vi "MPU_Stick_Plotter_Core.vi"(0 "Value (original)":dbl, 1 "Time (ms)":dbl, 2 "Offset & Multiplier":T2, 3 "Maximum":dbl, 4 "Minimum":dbl, 5 "error in (no error)":errorcluster, 6 "Channel Name":string, 7 "Plot update interval (ms)":u32=100, 8 "Number of vertical divisions":u16, 9 "Number of horizontal divisions":u16, 10 "Plot reference":refnum<vi>, 11 "Command":T3, 13 "Time axis length (ms)":u32=10000) -> (15 "Sample value":dbl, 16 "Plot Data":T1, 17 "Sample time (ms)":dbl, 19 "error out":errorcluster)   [LabVIEW 2017]
uses:
  Controls/MPU_Stick_Plotter_Core_Commands.ctl
  <vilib>/Utility/miscctls.llb/LVOffsetAndMultiplierTypeDef.ctl
  Controls/MPU_Stick_Plotter_Core_Channel_Data.ctl
  <vilib>/Utility/miscctls.llb/LVPointDoubleTypeDef.ctl
panel:
  in  "Use Internal timer ?":bool
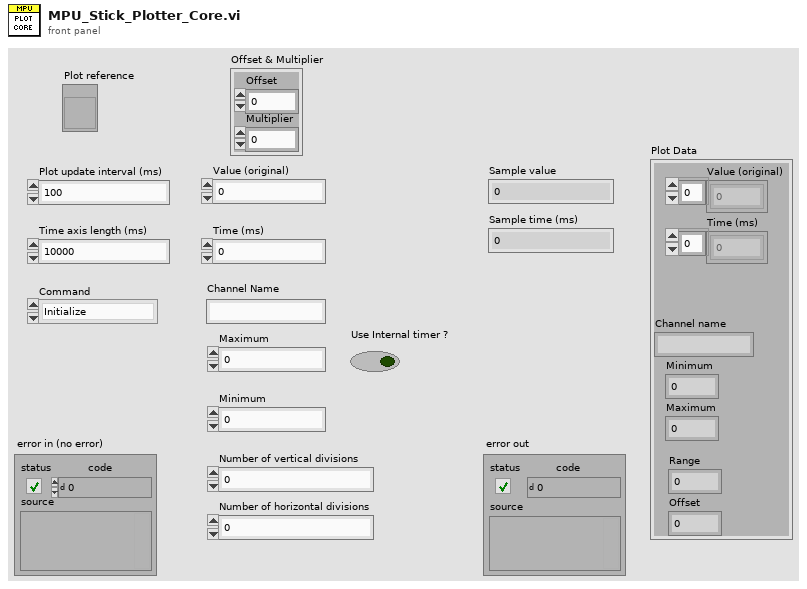
[diagram p1: front panel]
types:
  T1 = typedef "MPU_Stick_Plotter_Core_Channel_Data.ctl" = cluster{"Value (original)":dbl[], "Time (ms)":dbl[], "Channel name":string, "Minimum":dbl, "Maximum":dbl, "Offset":dbl, "Range":dbl}
  T2 = typedef "LVOffsetAndMultiplierTypeDef.ctl" = cluster{"Offset":dbl, "Multiplier":dbl}
  T3 = typedef "MPU_Stick_Plotter_Core_Commands.ctl" = enum16{"Initialize", "Add Channel", "Remove Channel", "Set Channel Minimum Value", "Set Channel Maximum Value", "Set Offset & Multiplier", "Get Offset & Multiplier", "Update Channel", "Get Cursor Data", "Clear", "Reset"}
  T4 = typedef "LVPointDoubleTypeDef.ctl" = cluster{"X":dbl, "Y":dbl}
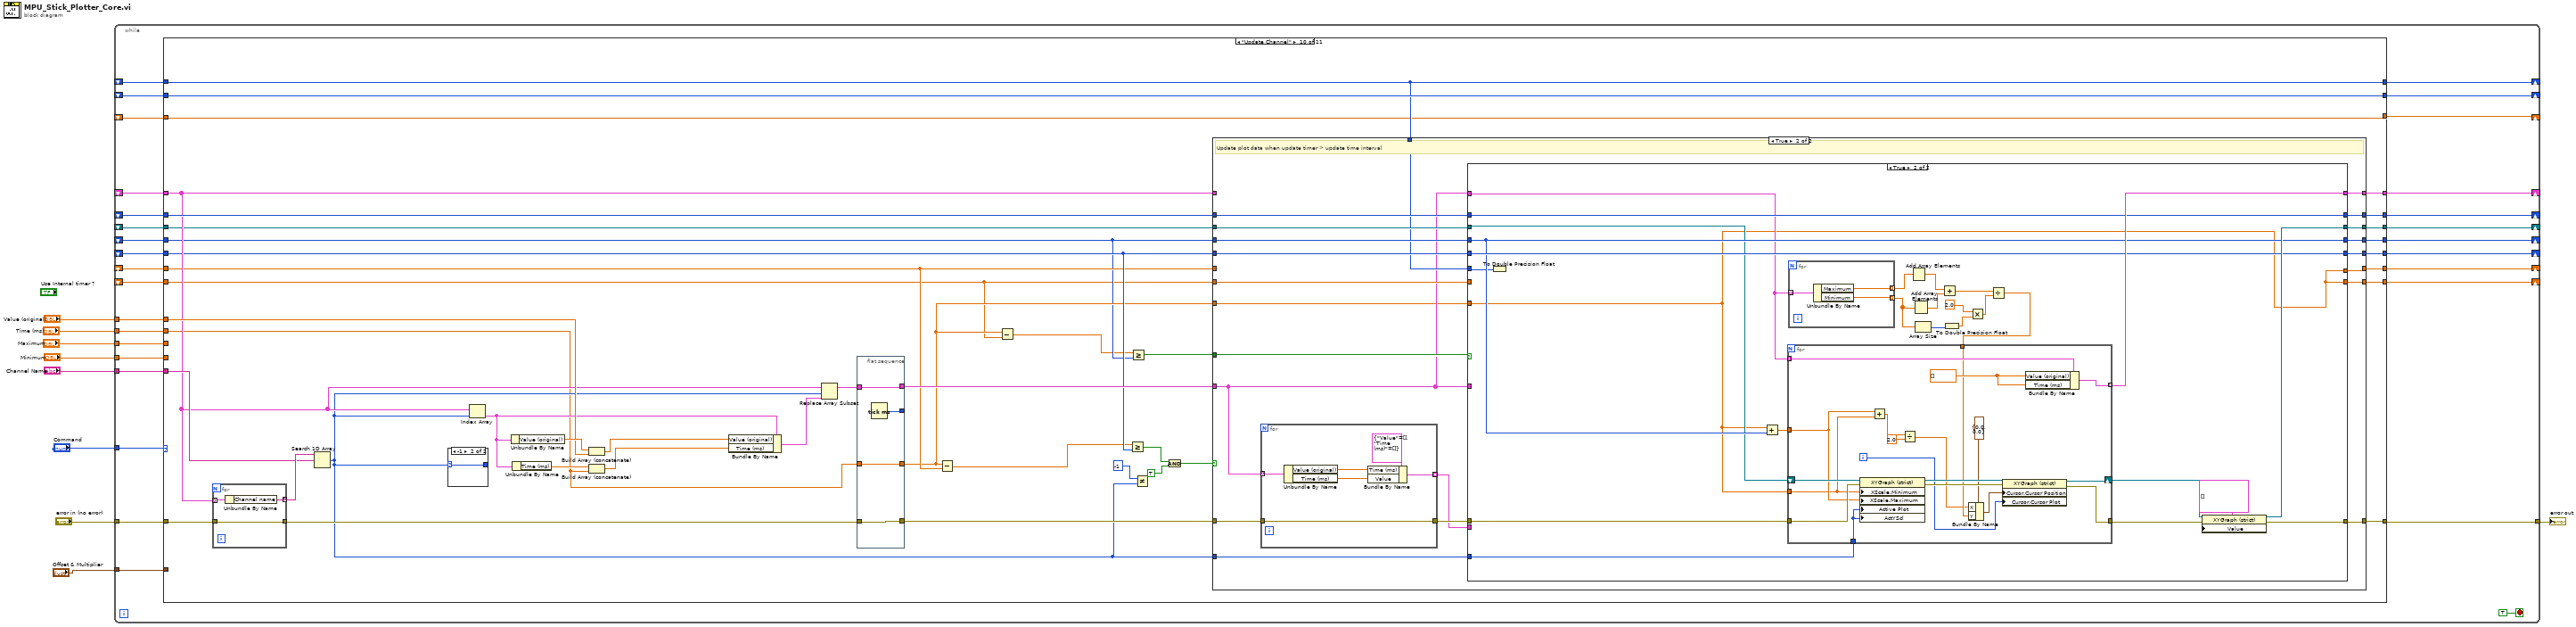
[diagram p0: block diagram]
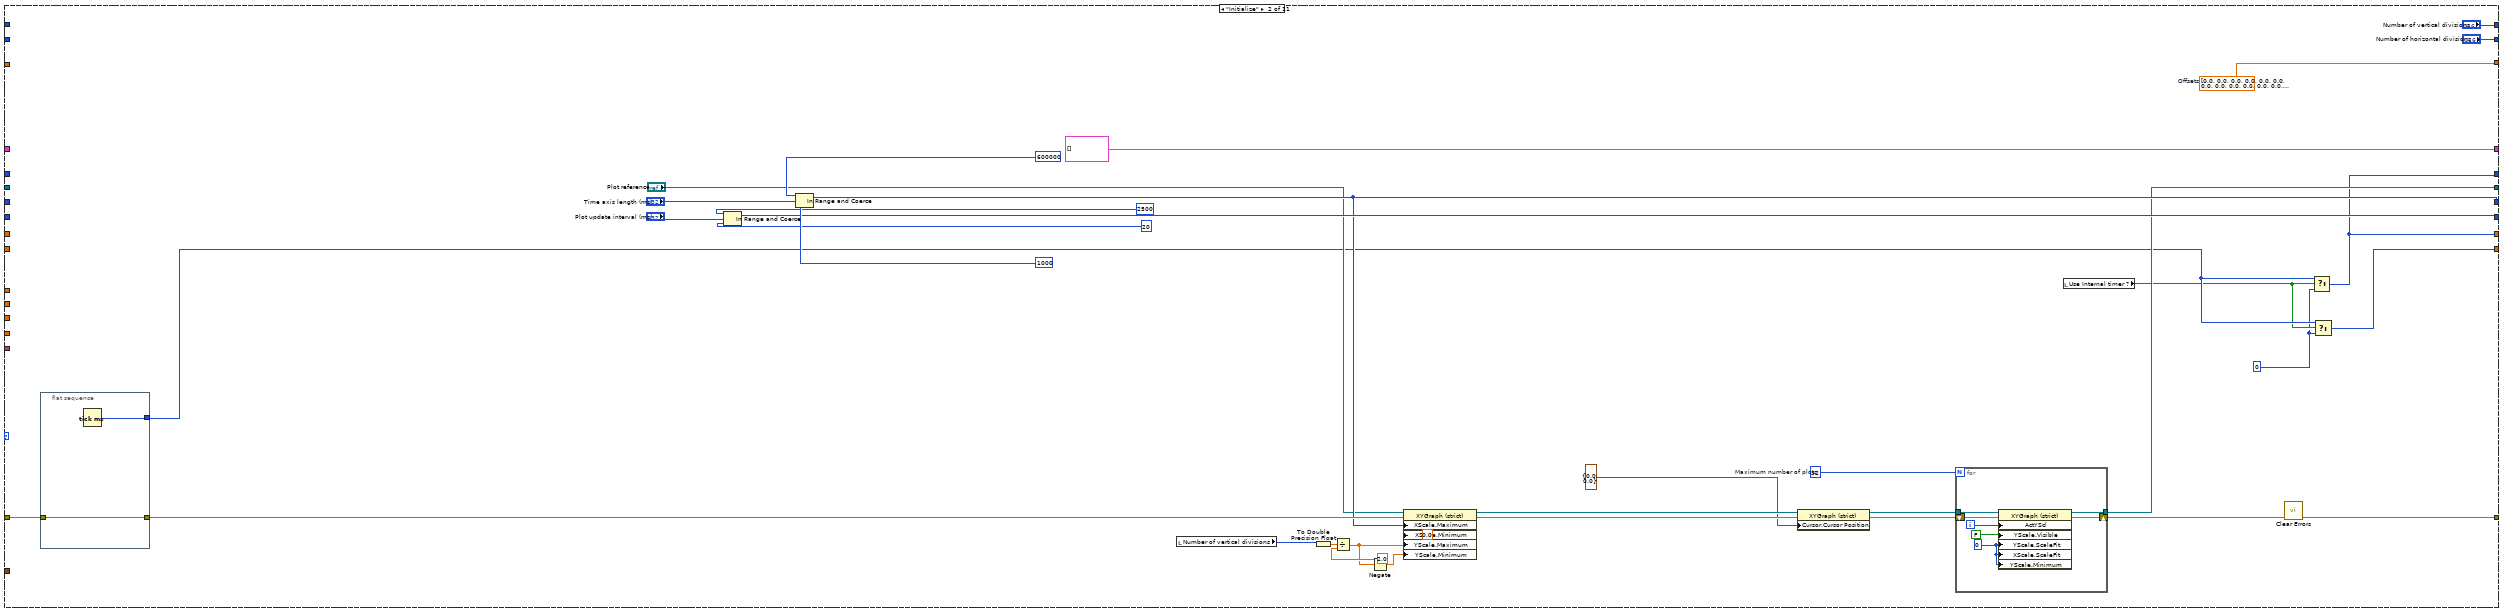
[diagram p3: hidden frame]
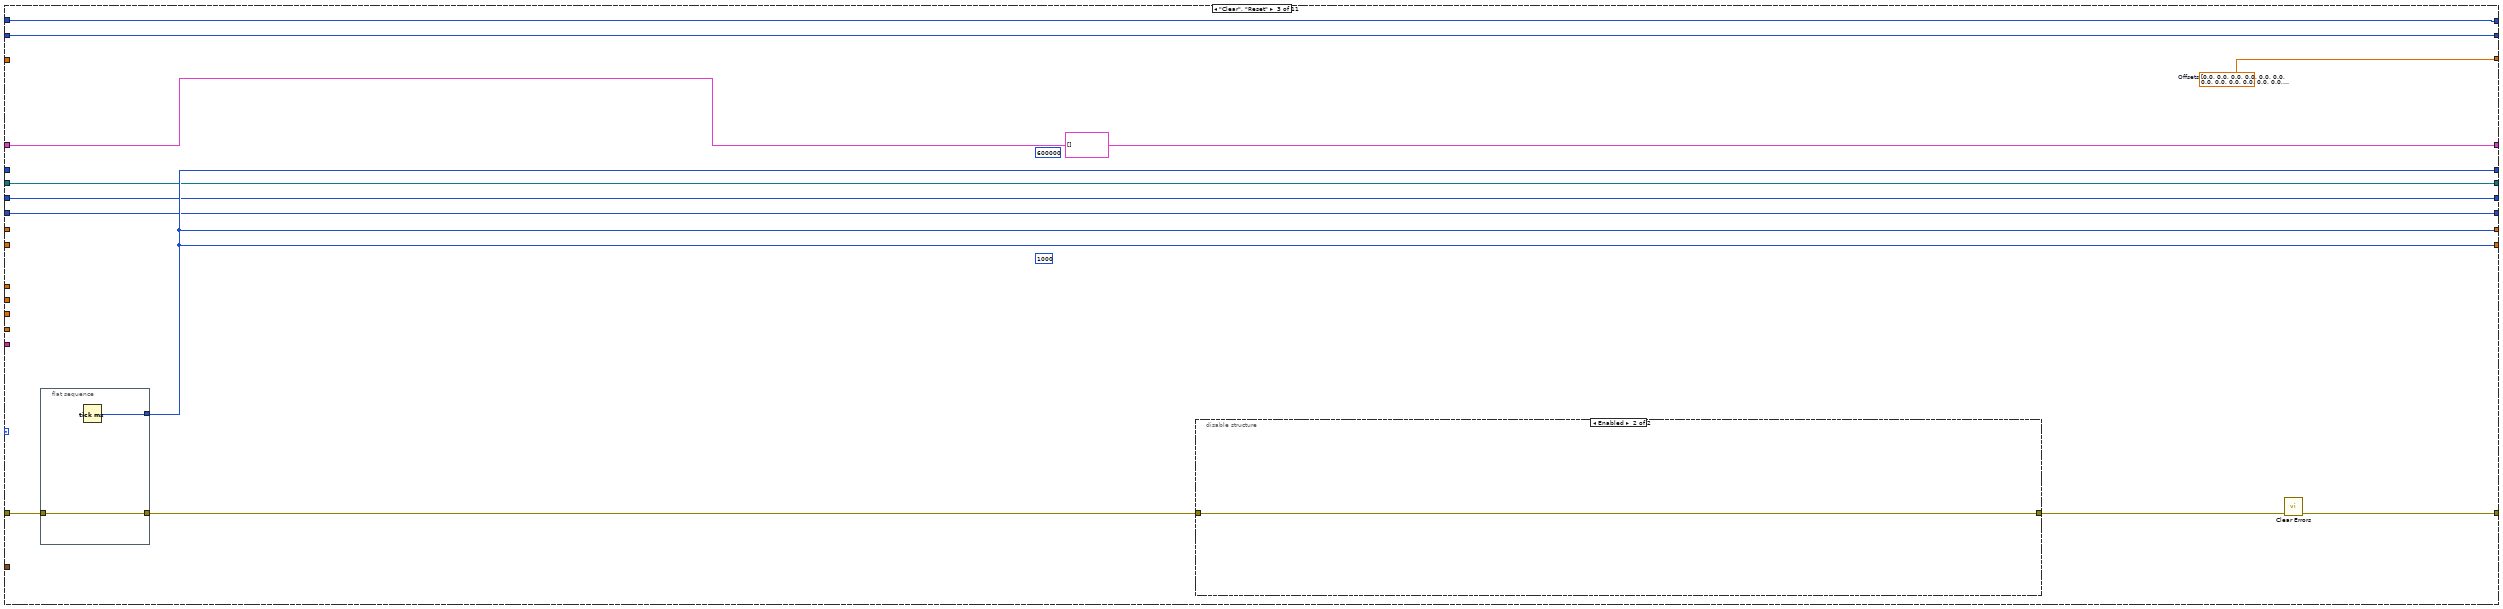
[diagram p4: hidden frame]
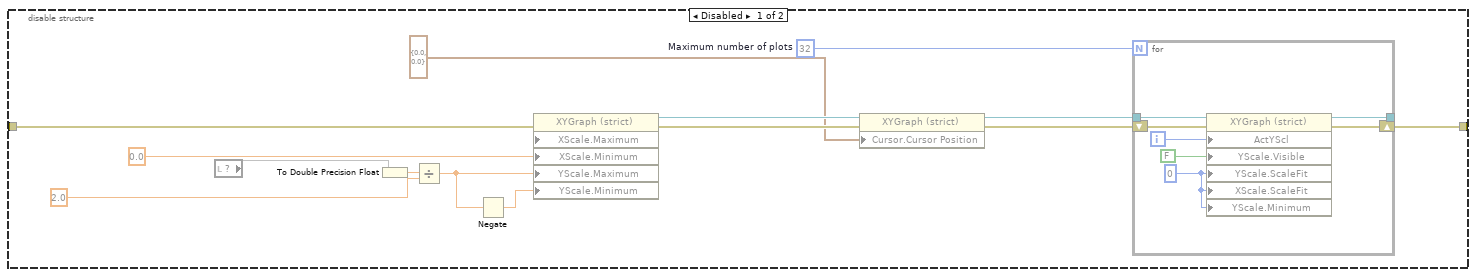
[diagram p5: hidden frame]
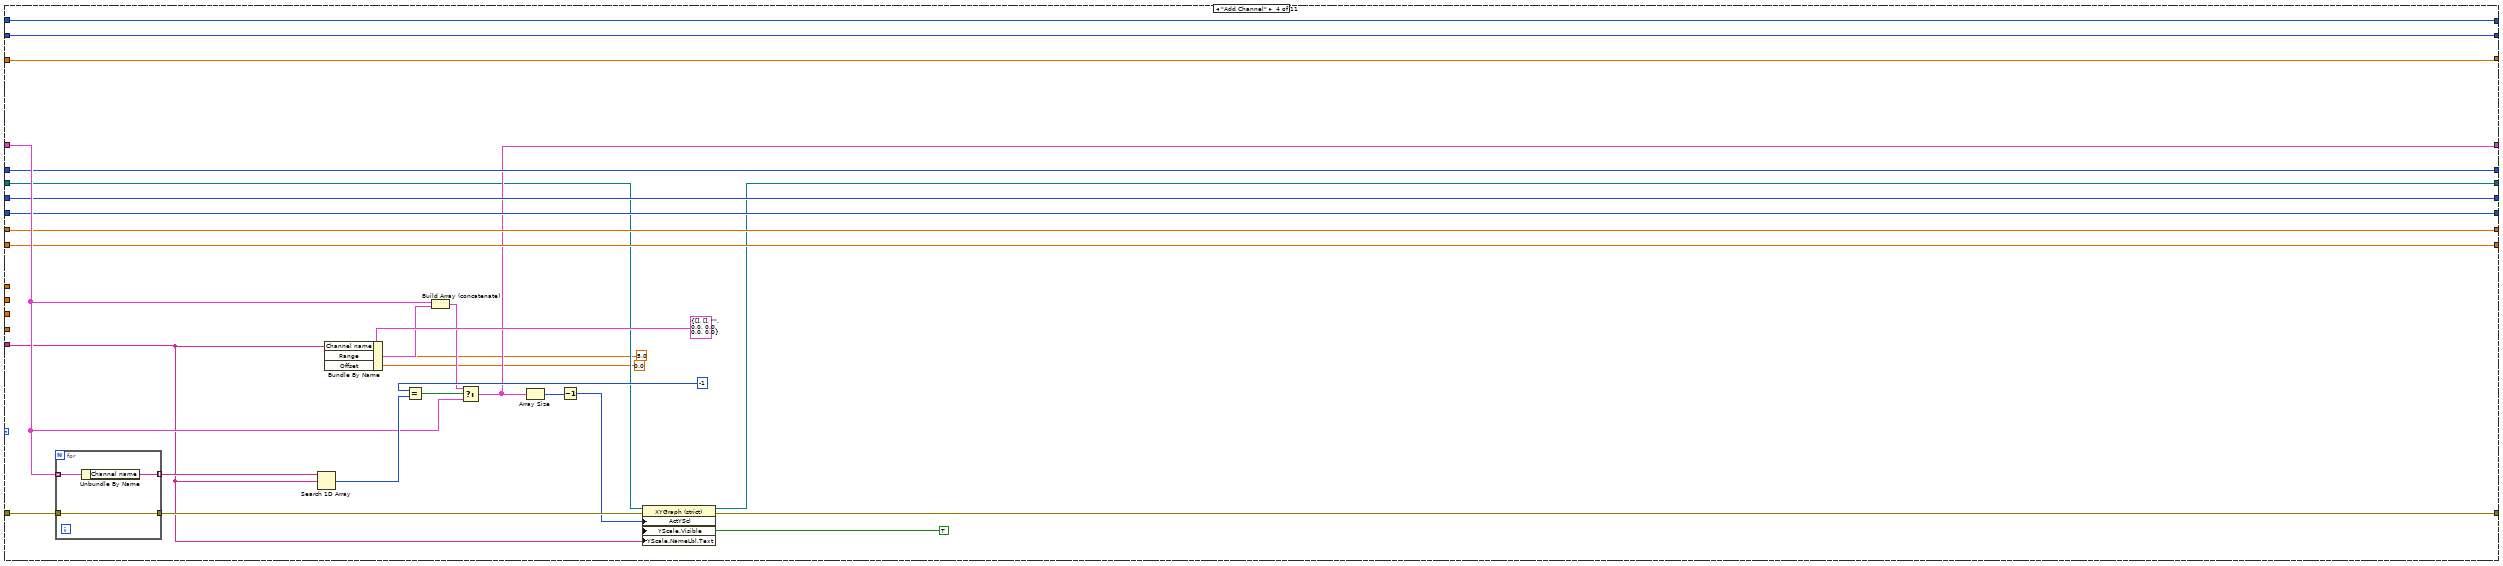
[diagram p6: hidden frame]
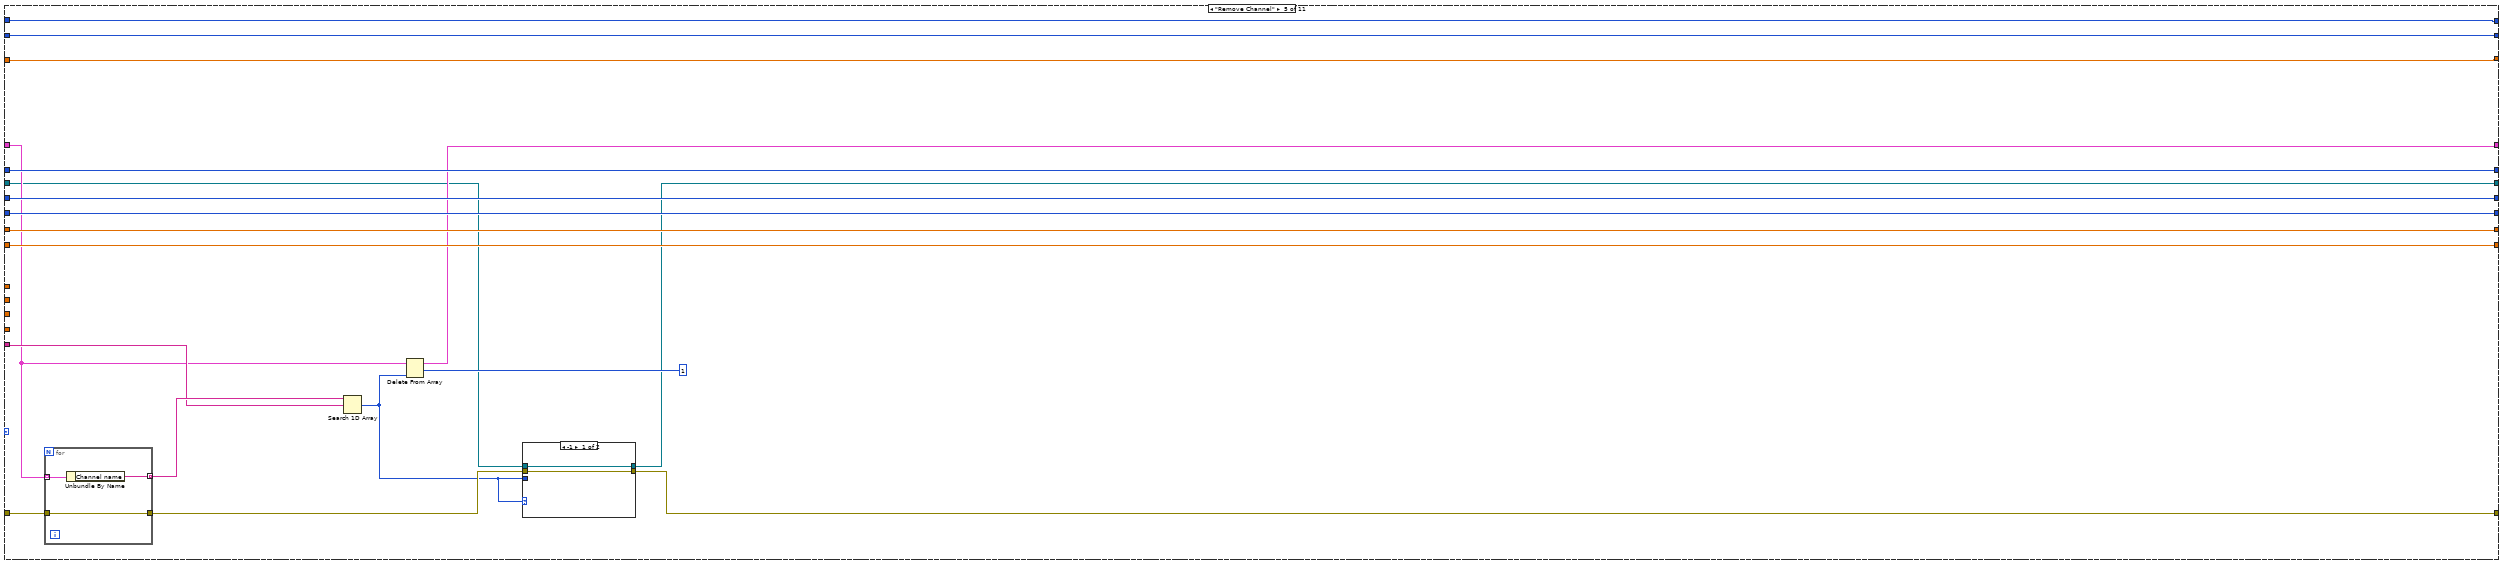
[diagram p7: hidden frame]
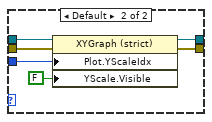
[diagram p8: hidden frame]
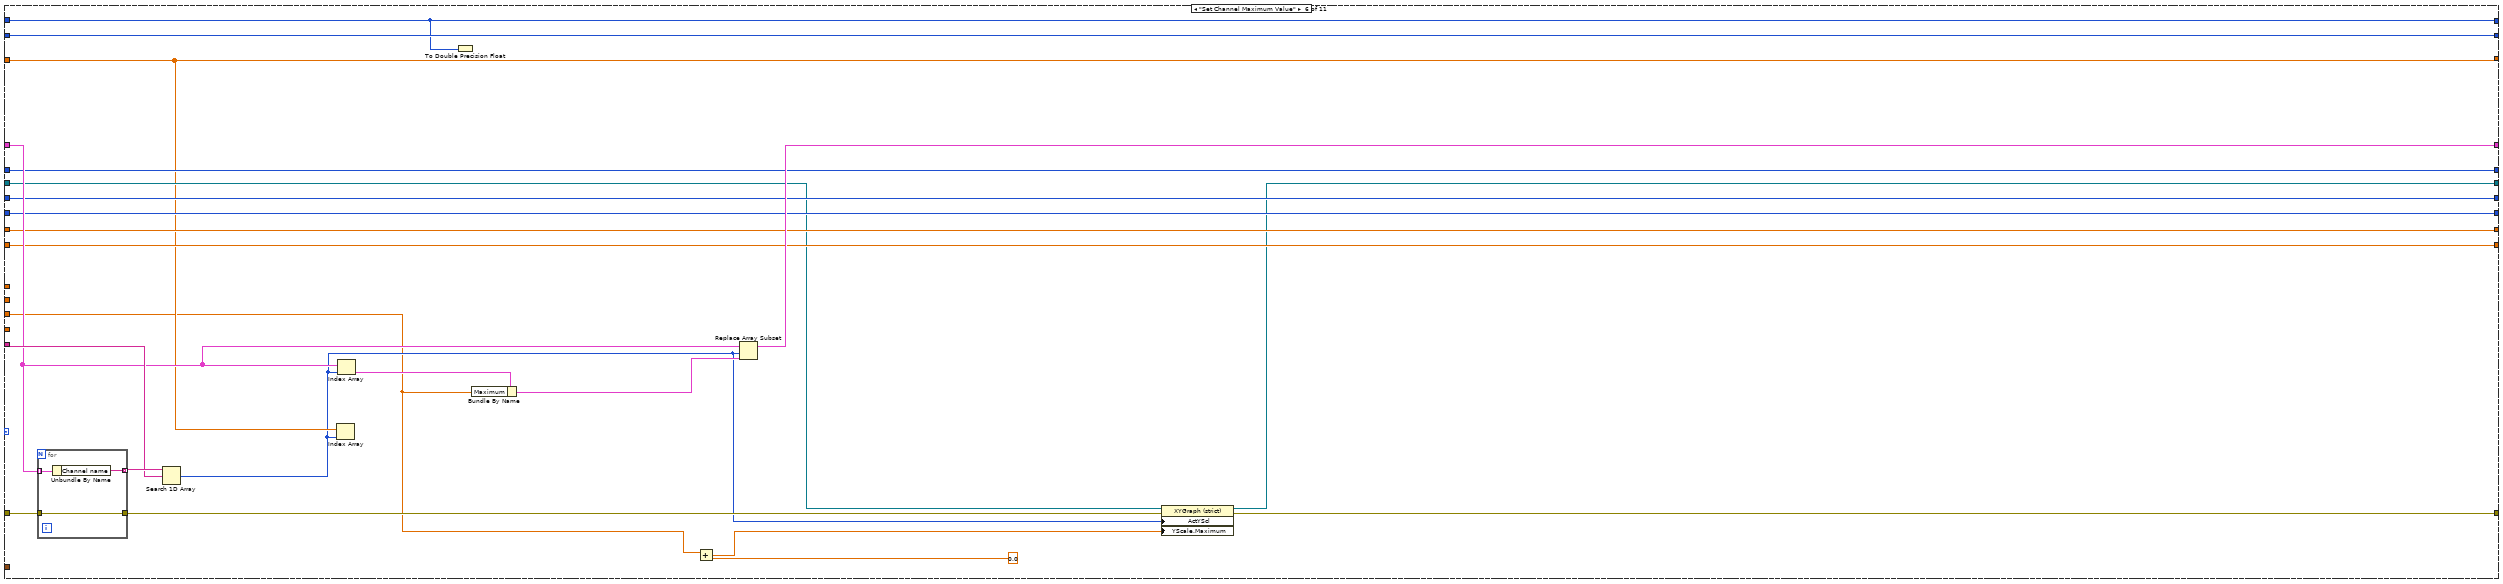
[diagram p9: hidden frame]
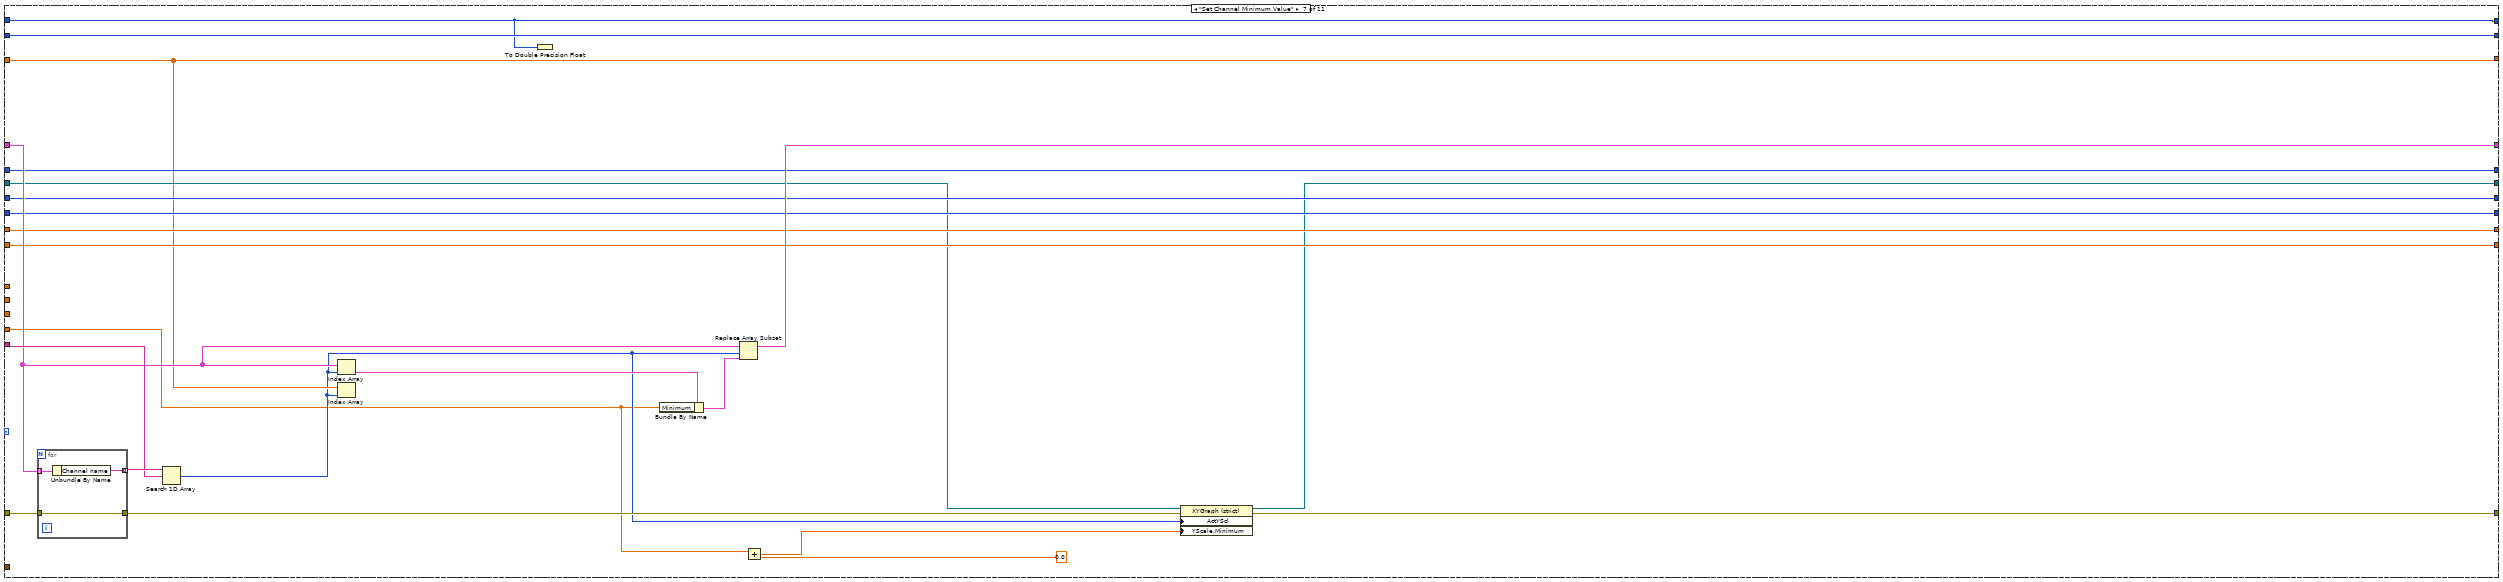
[diagram p10: hidden frame]
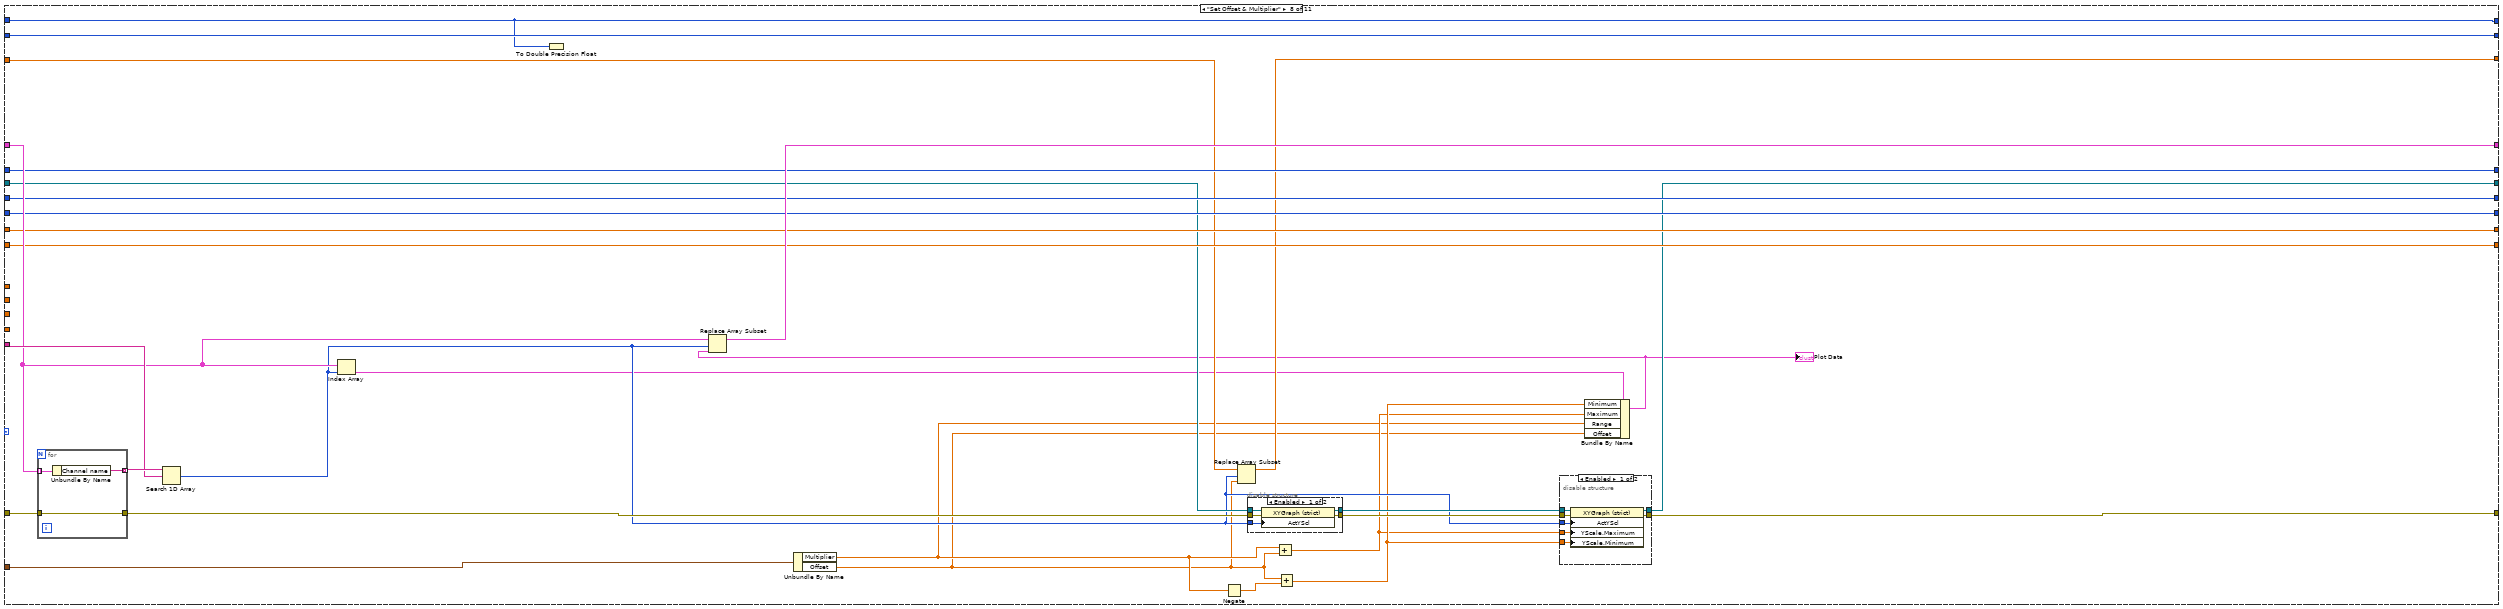
[diagram p11: hidden frame]
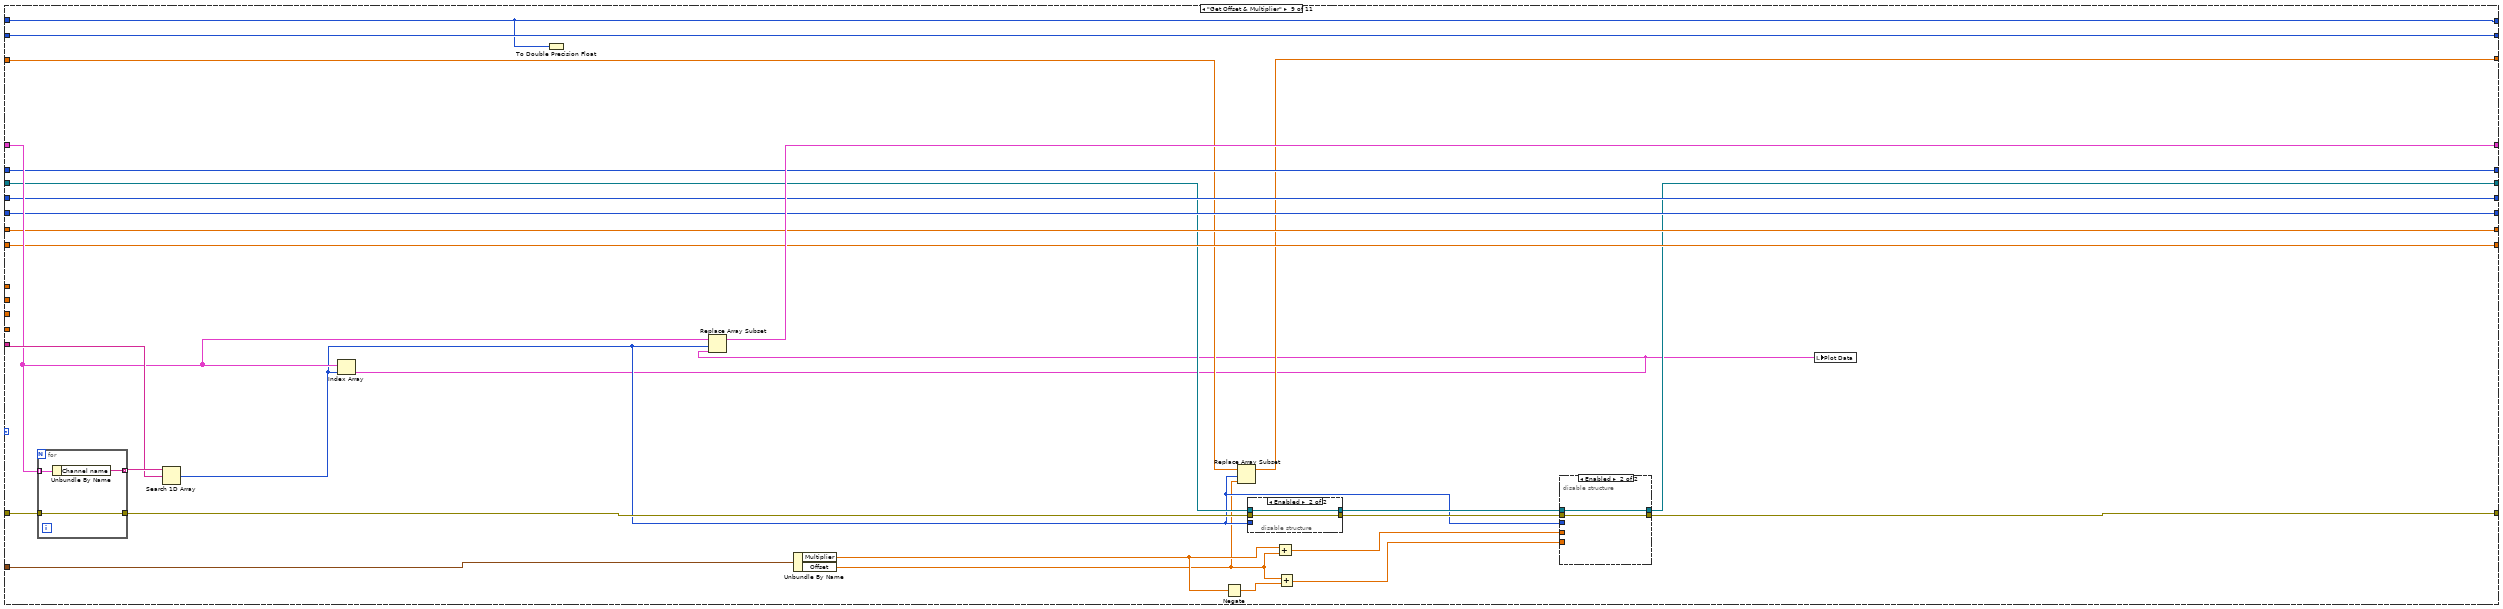
[diagram p14: hidden frame]
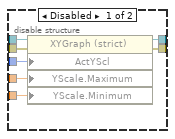
[diagram p15: hidden frame]
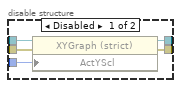
[diagram p16: hidden frame]
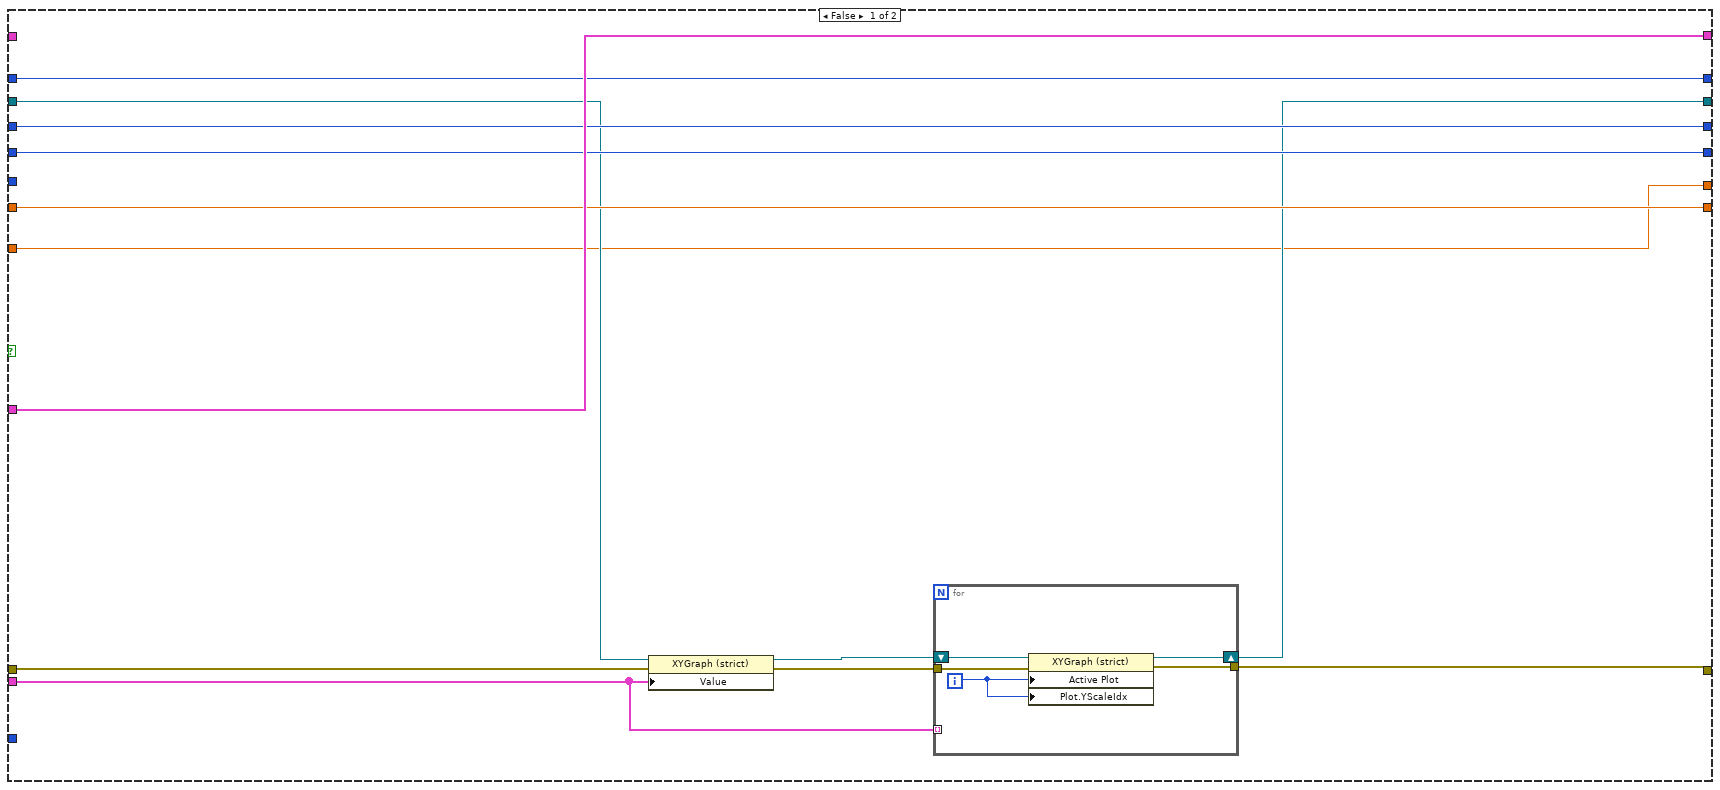
[diagram p19: hidden frame]
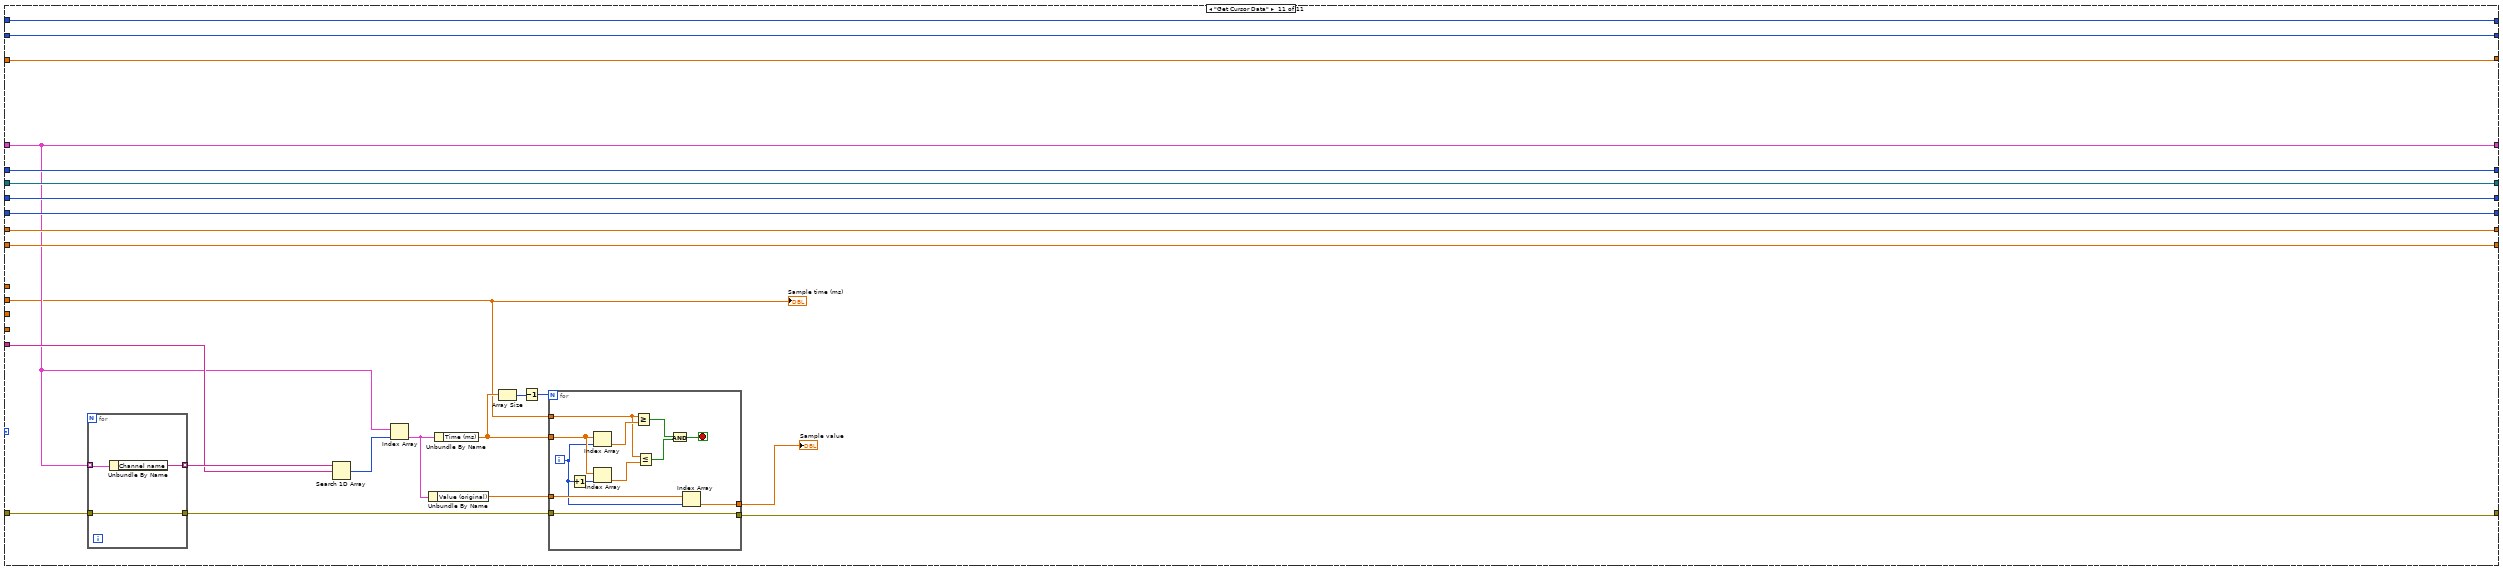
[diagram p20: hidden frame]
diagram:
  n1 = while {
    tunnel: "error in (no error)" -> [w37]
    tunnel: "Command" -> [w38]
    shift-right: [w36] -> _
    shift-left: _ -> [w35]
    tunnel: [w34] -> w7
    shift-right: [w33] -> _
    shift-left: _ -> [w32]
    shift-right: [w31] -> _
    shift-left: _ -> [w30]
    shift-right: [w29] -> _
    shift-left: _ -> [w27]
    shift-right: [w28] -> _
    shift-left: _ -> [w26]
    shift-right: [w25] -> _
    shift-left: _ -> [w23]
    shift-right: [w24] -> _
    shift-left: _ -> [w22]
    tunnel: "Value (original)" -> [w21]
    tunnel: "Time (ms)" -> [w20]
    tunnel: "Maximum" -> [w19]
    tunnel: "Minimum" -> [w18]
    tunnel: "Channel Name" -> [w17]
    shift-right: [w16] -> _
    shift-left: _ -> [w14]
    shift-right: [w15] -> _
    shift-left: _ -> [w13]
    tunnel: "Offset & Multiplier" -> [w12]
    shift-right: [w11] -> _
    shift-left: _ -> [w10]
    stop <- TRUE stop-if-true
    n2 = case shown="\"Update Channel\"" w38 {
      tunnel: w37 -> [w49 w84 w106 w159 w176 w215 w241 w273 w320 w381 w506]
      tunnel: [w50 T1[] [] w97 w141 w171 w211 w237 w269 w316 w372 w502] -> w36
      tunnel: w35 -> [w50 _ w97 w153 w173 w212 w238 w270 w317 w357 w502]
      tunnel: [w49 w56 w101 w142 w164 w203 w225 w258 w305 w365 w495] -> w34
      tunnel: [w48 w51 w105 w152 w181 w210 w235 w268 w315 w371 w512] -> w33
      tunnel: w32 -> [w48 _ _ w152 w181 w210 w235 w268 w315 w373 w512]
      tunnel: [w47 w59 w100 w135 w166 w198 w227 w255 w302 w370 w511] -> w31
      tunnel: w30 -> [w47 _ w100 w136 w167 w199 w228 w262 w309 w354 w511]
      tunnel: [w46 w72 w99 w151 w180 w209 w234 w267 w314 w369 w510] -> w29
      tunnel: [w45 w79 w98 w150 w179 w208 w233 w266 w313 w368 w509] -> w28
      tunnel: w27 -> [w46 _ w99 w151 w180 w209 w234 w267 w314 w342 w510]
      tunnel: w26 -> [w45 _ w98 w150 w179 w208 w233 w266 w313 w346 w509]
      tunnel: [w44 w51 w105 w149 w178 w207 w232 w265 w312 w366 w508] -> w25
      tunnel: [w43 w54 w105 w148 w177 w206 w231 w264 w311 w367 w507] -> w24
      tunnel: w23 -> [w44 _ _ w149 w178 w207 w232 w265 w312 w345 w508]
      tunnel: w22 -> [w43 _ _ w148 w177 w206 w231 w264 w311 w340 w507]
      tunnel: w21 -> [_ _ _ _ _ _ _ _ _ w377 _]
      tunnel: w20 -> [_ _ _ _ _ _ _ _ _ w347 w492]
      tunnel: w19 -> [_ _ _ _ _ w195 _ _ _ _ _]
      tunnel: w18 -> [_ _ _ _ _ _ w221 _ _ _ _]
      tunnel: w17 -> [_ _ _ w137 w174 w213 w239 w271 w318 w379 w504]
      tunnel: [w42 "Number of vertical divisions" w96 w147 w170 w202 w224 w260 w307 w360 w514] -> w16
      tunnel: [w41 "Number of horizontal divisions" w95 w146 w169 w205 w229 w263 w310 w361 w513] -> w15
      tunnel: w14 -> [w42 _ w96 w147 w170 w202 w224 w260 w307 w360 w514]
      tunnel: w13 -> [w41 _ w95 w146 w169 w205 w229 w263 w310 w361 w513]
      tunnel: w12 -> [_ _ _ _ _ _ _ w257 w304 _ _]
      tunnel: [w40 w58 w103 w134 w168 w197 w223 w254 w301 w353 w493] -> w11
      tunnel: w10 -> [w40 _ _ w134 w168 w197 w223 w253 w300 w353 w493]
      frame Default {
      }
      frame "Initialize" {
        w52 = u32 0 ("f")
        w58 = dbl[] [0.0, 0.0, 0.0, 0.0, 0.0, 0.0, 0.0, 0.0, 0.0, 0.0, 0.0, 0.0, 0.0, 0.0, 0.0, 0.0, 0.0, 0.0, 0.0, 0.0, 0.0, 0.0, 0.0, 0.0, 0.0, 0.0, 0.0, 0.0, 0.0, 0.0, 0.0, 0.0, 0.0, 0.0, 0.0, 0.0, 0.0, 0.0, 0.0, 0.0, 0.0, 0.0, 0.0, 0.0, 0.0, 0.0, 0.0, 0.0, 0.0, 0.0, 0.0, 0.0, 0.0, 0.0, 0.0, 0.0, 0.0, 0.0, 0.0, 0.0, 0.0, 0.0, 0.0, 0.0, 0.0, 0.0, 0.0, 0.0, 0.0, 0.0, 0.0, 0.0, 0.0, 0.0, 0.0, 0.0, 0.0, 0.0, 0.0, 0.0, 0.0, 0.0, 0.0, 0.0, 0.0, 0.0, 0.0, 0.0, 0.0, 0.0, 0.0, 0.0, 0.0, 0.0, 0.0, 0.0, 0.0, 0.0, 0.0, 0.0, 0.0, 0.0, 0.0, 0.0, 0.0, 0.0, 0.0, 0.0, 0.0, 0.0, 0.0, 0.0, 0.0, 0.0, 0.0, 0.0, 0.0, 0.0, 0.0, 0.0, 0.0, 0.0, 0.0, 0.0, 0.0, 0.0, 0.0, 0.0, 0.0, 0.0, 0.0, 0.0, 0.0, 0.0, 0.0, 0.0, 0.0, 0.0, 0.0, 0.0, 0.0, 0.0, 0.0, 0.0, 0.0, 0.0, 0.0, 0.0, 0.0, 0.0, 0.0, 0.0, 0.0, 0.0, 0.0, 0.0, 0.0, 0.0, 0.0, 0.0, 0.0, 0.0, 0.0, 0.0, 0.0, 0.0, 0.0, 0.0, 0.0, 0.0, 0.0, 0.0, 0.0, 0.0, 0.0, 0.0, 0.0, 0.0, 0.0, 0.0, 0.0, 0.0, 0.0, 0.0, 0.0, 0.0, 0.0, 0.0, 0.0, 0.0, 0.0, 0.0, 0.0, 0.0, 0.0, 0.0, 0.0, 0.0, 0.0, 0.0, 0.0, 0.0, 0.0, 0.0, 0.0, 0.0, 0.0, 0.0, 0.0, 0.0, 0.0, 0.0, 0.0, 0.0, 0.0, 0.0, 0.0, 0.0, 0.0, 0.0, 0.0, 0.0, 0.0, 0.0, 0.0, 0.0, 0.0, 0.0, 0.0, 0.0, 0.0, 0.0, 0.0, 0.0, 0.0, 0.0, 0.0, 0.0, 0.0, 0.0, 0.0, 0.0, 0.0, 0.0, 0.0, 0.0, 0.0, 0.0, 0.0, 0.0, 0.0, 0.0, 0.0, 0.0, 0.0, 0.0]  # Offsets
        w61 = 32  # Maximum number of plots
        n3 = flat-sequence {
          tunnel: w84 -> [w94]
          tunnel: [w94] -> w73
          tunnel: [w93] -> w55
          frame #0 {
            n4 = Tick Count (ms)() -> (millisecond timer value=w93:u32)
          }
        }
        n5 = In Range and Coerce(upper limit=u32 2500, x="Plot update interval (ms)", lower limit=u32 20) -> (coerced(x)=w79:u32)  [unwired: 1 out]
        n6 = In Range and Coerce(upper limit=u32 600000, x="Time axis length (ms)", lower limit=u32 1000) -> (coerced(x)=w72:u32)  [unwired: 1 out]
        n7 = local read "Number of vertical divisions"() -> (w67:u16)
        n8 = To Double Precision Float(number=w67) -> (double precision float=w71:dbl)
        n9 = Divide(x=w71, y=2.0) -> (x/y=w69:dbl)
        n10 = Negate(x=w69) -> (-x=w68:dbl)
        n11 = property class="XYGraph (strict)"(reference="Plot reference", error in=w73, "XScale.Maximum"=w72, "XScale.Minimum"=0.0 ("X Scale.Range:Minimum"), "YScale.Maximum"=w69, "YScale.Minimum"=w68) -> (reference out=w65:refnum<vi>, error out=w66:errorcluster)
        n12 = property class="XYGraph (strict)"(reference=w65, error in=w66, "Cursor.Cursor Position"=T4 {"X"=0.0, "Y"=0.0}) -> (reference out=w63:refnum<vi>, error out=w62:errorcluster)
        n13 = for {
          N: w61 -> [_]
          tunnel: w63 -> [w92]
          shift-right: [w90] -> w57
          shift-left: w62 -> [w91]
          tunnel: [w87] -> w59
          i -> [w89]
          w86 = u8 0 ("Y Scale.Scale Fit")
          n14 = property class="XYGraph (strict)"(reference=w92, error in=w91, "ActYScl"=w89, "YScale.Visible"=FALSE ("Y Scale.Visible"), "YScale.ScaleFit"=w86, "XScale.ScaleFit"=w86, "YScale.Minimum"=w86) -> (reference out=w87:refnum<vi>, error out=w90:errorcluster)
        }
        n15 = local read "Use Internal timer ?"() -> (w53:bool)
        n16 = call <vilib>:"Clear Errors.vi"("error in (no error)"=w57) -> ("error out"=w56:errorcluster)  [unwired: 5 in, 1 out]
        n17 = Select(t=w55, s=w53, f=w52) -> (s? t:f=w51:u32)
        n18 = Select(t=w55, s=w53, f=w52) -> (s? t:f=w54:u32)
      }
      frame "Clear", "Reset" {
        w103 = dbl[] [0.0, 0.0, 0.0, 0.0, 0.0, 0.0, 0.0, 0.0, 0.0, 0.0, 0.0, 0.0, 0.0, 0.0, 0.0, 0.0, 0.0, 0.0, 0.0, 0.0, 0.0, 0.0, 0.0, 0.0, 0.0, 0.0, 0.0, 0.0, 0.0, 0.0, 0.0, 0.0, 0.0, 0.0, 0.0, 0.0, 0.0, 0.0, 0.0, 0.0, 0.0, 0.0, 0.0, 0.0, 0.0, 0.0, 0.0, 0.0, 0.0, 0.0, 0.0, 0.0, 0.0, 0.0, 0.0, 0.0, 0.0, 0.0, 0.0, 0.0, 0.0, 0.0, 0.0, 0.0, 0.0, 0.0, 0.0, 0.0, 0.0, 0.0, 0.0, 0.0, 0.0, 0.0, 0.0, 0.0, 0.0, 0.0, 0.0, 0.0, 0.0, 0.0, 0.0, 0.0, 0.0, 0.0, 0.0, 0.0, 0.0, 0.0, 0.0, 0.0, 0.0, 0.0, 0.0, 0.0, 0.0, 0.0, 0.0, 0.0, 0.0, 0.0, 0.0, 0.0, 0.0, 0.0, 0.0, 0.0, 0.0, 0.0, 0.0, 0.0, 0.0, 0.0, 0.0, 0.0, 0.0, 0.0, 0.0, 0.0, 0.0, 0.0, 0.0, 0.0, 0.0, 0.0, 0.0, 0.0, 0.0, 0.0, 0.0, 0.0, 0.0, 0.0, 0.0, 0.0, 0.0, 0.0, 0.0, 0.0, 0.0, 0.0, 0.0, 0.0, 0.0, 0.0, 0.0, 0.0, 0.0, 0.0, 0.0, 0.0, 0.0, 0.0, 0.0, 0.0, 0.0, 0.0, 0.0, 0.0, 0.0, 0.0, 0.0, 0.0, 0.0, 0.0, 0.0, 0.0, 0.0, 0.0, 0.0, 0.0, 0.0, 0.0, 0.0, 0.0, 0.0, 0.0, 0.0, 0.0, 0.0, 0.0, 0.0, 0.0, 0.0, 0.0, 0.0, 0.0, 0.0, 0.0, 0.0, 0.0, 0.0, 0.0, 0.0, 0.0, 0.0, 0.0, 0.0, 0.0, 0.0, 0.0, 0.0, 0.0, 0.0, 0.0, 0.0, 0.0, 0.0, 0.0, 0.0, 0.0, 0.0, 0.0, 0.0, 0.0, 0.0, 0.0, 0.0, 0.0, 0.0, 0.0, 0.0, 0.0, 0.0, 0.0, 0.0, 0.0, 0.0, 0.0, 0.0, 0.0, 0.0, 0.0, 0.0, 0.0, 0.0, 0.0, 0.0, 0.0, 0.0, 0.0, 0.0, 0.0, 0.0, 0.0, 0.0, 0.0, 0.0, 0.0, 0.0, 0.0, 0.0, 0.0, 0.0, 0.0]  # Offsets
        (unwired) u32 1000 ("lower limit")
        (unwired) u32 600000 ("upper limit")
        (unwired) T1[] []
        n19 = flat-sequence {
          tunnel: w106 -> [w131]
          tunnel: [w131] -> w104
          tunnel: [w130] -> w105
          frame #0 {
            n20 = Tick Count (ms)() -> (millisecond timer value=w130:u32)
          }
        }
        n21 = disable-structure shown="Enabled" {
          disable-tunnel: w104 -> [w120 w129]
          disable-tunnel: [w108 w129] -> w102
          frame Disabled {
            w109 = 32  # Maximum number of plots
            n22 = local read item#-1() -> (w115)
            n23 = To Double Precision Float(number=w115) -> (double precision float=w119:dbl)
            n24 = Divide(x=w119, y=2.0) -> (x/y=w117:dbl)
            n25 = Negate(x=w117) -> (-x=w116:dbl)
            n26 = property class="XYGraph (strict)" props=["XScale", "Maximum", "XScale", "Minimum", "YScale", "Maximum", "YScale", "Minimum"](error in=w120, "XScale.Minimum"=0.0 ("X Scale.Range:Minimum"), "YScale.Maximum"=w117, "YScale.Minimum"=w116) -> (reference out=w113:refnum<vi>, error out=w114:errorcluster)  [unwired: 2 in]
            n27 = property class="XYGraph (strict)"(reference=w113, error in=w114, "Cursor.Cursor Position"=T4 {"X"=0.0, "Y"=0.0}) -> (reference out=w111:refnum<vi>, error out=w110:errorcluster)
            n28 = for {
              N: w109 -> [_]
              tunnel: w111 -> [w128]
              shift-right: [w126] -> w108
              shift-left: w110 -> [w127]
              tunnel: [w123] -> w107
              i -> [w125]
              w122 = u8 0 ("Y Scale.Scale Fit")
              n29 = property class="XYGraph (strict)"(reference=w128, error in=w127, "ActYScl"=w125, "YScale.Visible"=FALSE ("Y Scale.Visible"), "YScale.ScaleFit"=w122, "XScale.ScaleFit"=w122, "YScale.Minimum"=w122) -> (reference out=w123:refnum<vi>, error out=w126:errorcluster)
            }
          }
          frame Enabled {
          }
        }
        n30 = call <vilib>:"Clear Errors.vi"("error in (no error)"=w102) -> ("error out"=w101:errorcluster)  [unwired: 5 in, 1 out]
      }
      frame "Add Channel" {
        n31 = for {
          tunnel: w159 -> [w161]
          tunnel: w153 -> [w162] mode=indexing
          tunnel: [w161] -> w143
          tunnel: [w160] -> w158 mode=indexing
          n32 = Unbundle By Name(w162) -> ("Channel name"=w160:string)
        }
        n33 = Search 1D Array(1D array=w158, element=w137) -> (index of element=w157:i32)  [unwired: 1 in]
        n34 = Bundle By Name(cluster=T1 {"Value (original)"=[], "Time (ms)"=[], "Channel name"="", "Minimum"=0.0, "Maximum"=0.0, "Offset"=0.0, "Range"=0.0} ("Plotter_Channel_Data"), "Channel name"=w137, "Range"=5.0, "Offset"=0.0 ("Maximum")) -> (w145:T1)
        n35 = Equal?(x=-1, y=w157) -> (x = y?=w155:bool)
        n36 = Build Array (concatenate)(w153, w145) -> (w144:T1[])
        n37 = Select(t=w144, s=w155, f=w153) -> (s? t:f=w141:T1[])
        n38 = Array Size(array=w141) -> (size(s)=w140:i32)
        n39 = Decrement(x=w140) -> (x-1=w139:i32)
        n40 = property class="XYGraph (strict)"(reference=w136, error in=w143, "ActYScl"=w139, "YScale.Visible"=TRUE ("Y Scale.Visible"), "YScale.NameLbl.Text"=w137) -> (reference out=w135:refnum<vi>, error out=w142:errorcluster)
      }
      frame "Remove Channel" {
        n41 = for {
          tunnel: w176 -> [w192]
          tunnel: [w192] -> w165
          tunnel: w173 -> [w191] mode=indexing
          tunnel: [w190] -> w175 mode=indexing
          n42 = Unbundle By Name(w191) -> ("Channel name"=w190:string)
        }
        n43 = Search 1D Array(1D array=w175, element=w174) -> (index of element=w163:i32)  [unwired: 1 in]
        n44 = Delete From Array(array=w173, length=1, index=w163) -> (array with subset deleted=w171:T1[])  [unwired: 1 out]
        n45 = case shown="-1" w163 {
          tunnel: w167 -> [w183 w189]
          tunnel: [w183 w188] -> w166
          tunnel: w165 -> [w182 w187]
          tunnel: [w182 w186] -> w164
          tunnel: w163 -> [_ w184]
          frame -1 {
          }
          frame Default {
            n46 = property class="XYGraph (strict)"(reference=w189, error in=w187, "Plot.YScaleIdx"=w184, "YScale.Visible"=FALSE ("Y Scale.Visible")) -> (reference out=w188:refnum<vi>, error out=w186:errorcluster)
          }
        }
      }
      frame "Set Channel Maximum Value" {
        n47 = for {
          tunnel: w215 -> [w218]
          tunnel: [w218] -> w204
          tunnel: w212 -> [w217] mode=indexing
          tunnel: [w216] -> w214 mode=indexing
          n48 = Unbundle By Name(w217) -> ("Channel name"=w216:string)
        }
        n49 = Search 1D Array(1D array=w214, element=w213) -> (index of element=w196:i32)  [unwired: 1 in]
        n50 = Index Array(array=w197, index=w196) -> ()  [unwired: 1 out]
        n51 = Index Array(array=w212, index=w196) -> (element=w201:T1)
        n52 = To Double Precision Float(number=w202) -> ()  [unwired: 1 out]
        n53 = Bundle By Name(cluster=w201, "Maximum"=w195) -> (w200:T1)
        n54 = Add(x=w195, y=0.0) -> (x+y=w194:dbl)
        n55 = Replace Array Subset(array=w212, new element=w200, index=w196) -> (w211:T1[])
        n56 = property class="XYGraph (strict)"(reference=w199, error in=w204, "ActYScl"=w196, "YScale.Maximum"=w194) -> (reference out=w198:refnum<vi>, error out=w203:errorcluster)
      }
      frame "Set Channel Minimum Value" {
        n57 = for {
          tunnel: w241 -> [w244]
          tunnel: [w244] -> w226
          tunnel: w238 -> [w243] mode=indexing
          tunnel: [w242] -> w240 mode=indexing
          n58 = Unbundle By Name(w243) -> ("Channel name"=w242:string)
        }
        n59 = Search 1D Array(1D array=w240, element=w239) -> (index of element=w222:i32)  [unwired: 1 in]
        n60 = Index Array(array=w238, index=w222) -> (element=w230:T1)
        n61 = Index Array(array=w223, index=w222) -> ()  [unwired: 1 out]
        n62 = To Double Precision Float(number=w224) -> ()  [unwired: 1 out]
        n63 = Bundle By Name(cluster=w230, "Minimum"=w221) -> (w236:T1)
        n64 = Replace Array Subset(array=w238, new element=w236, index=w222) -> (w237:T1[])
        n65 = Add(x=w221, y=0.0) -> (x+y=w220:dbl)
        n66 = property class="XYGraph (strict)"(reference=w228, error in=w226, "ActYScl"=w222, "YScale.Minimum"=w220) -> (reference out=w227:refnum<vi>, error out=w225:errorcluster)
      }
      frame "Set Offset & Multiplier" {
        n67 = for {
          tunnel: w273 -> [w292]
          tunnel: [w292] -> w261
          tunnel: w270 -> [w291] mode=indexing
          tunnel: [w290] -> w272 mode=indexing
          n68 = Unbundle By Name(w291) -> ("Channel name"=w290:string)
        }
        n69 = Search 1D Array(1D array=w272, element=w271) -> (index of element=w252:i32)  [unwired: 1 in]
        n70 = Index Array(array=w270, index=w252) -> (element=w251:T1)
        n71 = To Double Precision Float(number=w260) -> ()  [unwired: 1 out]
        n72 = Unbundle By Name(w257) -> ("Multiplier"=w246:dbl, "Offset"=w245:dbl)
        n73 = Negate(x=w246) -> (-x=w249:dbl)
        n74 = Replace Array Subset(array=w253, new element=w245, index=w252) -> (w254:dbl[])
        n75 = disable-structure shown="Enabled" {
          disable-tunnel: w262 -> [w287 w289]
          disable-tunnel: w261 -> [w286 w288]
          disable-tunnel: [w285 w288] -> w259
          disable-tunnel: [w284 w289] -> w256
          disable-tunnel: w252 -> [w283 _]
          frame Enabled {
            n76 = property class="XYGraph (strict)"(reference=w287, error in=w286, "ActYScl"=w283) -> (reference out=w284:refnum<vi>, error out=w285:errorcluster)
          }
          frame Disabled {
          }
        }
        n77 = Add(x=w246, y=w245) -> (x+y=w247:dbl)
        n78 = Add(x=w245, y=w249) -> (x+y=w248:dbl)
        n79 = disable-structure shown="Enabled" {
          disable-tunnel: w259 -> [w280 w281]
          disable-tunnel: [w279 w281] -> w258
          disable-tunnel: w252 -> [w278 _]
          disable-tunnel: w256 -> [w277 w282]
          disable-tunnel: [w276 w282] -> w255
          disable-tunnel: w247 -> [w275 _]
          disable-tunnel: w248 -> [w274 _]
          frame Enabled {
            n80 = property class="XYGraph (strict)"(reference=w277, error in=w280, "ActYScl"=w278, "YScale.Maximum"=w275, "YScale.Minimum"=w274) -> (reference out=w276:refnum<vi>, error out=w279:errorcluster)
          }
          frame Disabled {
          }
        }
        n81 = Bundle By Name(cluster=w251, "Minimum"=w248, "Maximum"=w247, "Range"=w246, "Offset"=w245) -> (w250:T1)
        "Plot Data" <- w250
        n82 = Replace Array Subset(array=w270, new element=w250, index=w252) -> (w269:T1[])
      }
      frame "Get Offset & Multiplier" {
        n83 = for {
          tunnel: w320 -> [w339]
          tunnel: [w339] -> w308
          tunnel: w317 -> [w338] mode=indexing
          tunnel: [w337] -> w319 mode=indexing
          n84 = Unbundle By Name(w338) -> ("Channel name"=w337:string)
        }
        n85 = Search 1D Array(1D array=w319, element=w318) -> (index of element=w299:i32)  [unwired: 1 in]
        n86 = Index Array(array=w317, index=w299) -> (element=w293:T1)
        n87 = To Double Precision Float(number=w307) -> ()  [unwired: 1 out]
        n88 = Replace Array Subset(array=w317, new element=w293, index=w299) -> (w316:T1[])
        n89 = Unbundle By Name(w304) -> ("Multiplier"=w295:dbl, "Offset"=w294:dbl)
        n90 = Negate(x=w295) -> (-x=w298:dbl)
        n91 = Replace Array Subset(array=w300, new element=w294, index=w299) -> (w301:dbl[])
        n92 = disable-structure shown="Enabled" {
          disable-tunnel: w309 -> [w334 w336]
          disable-tunnel: w308 -> [w333 w335]
          disable-tunnel: [w332 w335] -> w306
          disable-tunnel: [w331 w336] -> w303
          disable-tunnel: w299 -> [w330 _]
          frame Disabled {
            n93 = property class="XYGraph (strict)"(reference=w334, error in=w333, "ActYScl"=w330) -> (reference out=w331:refnum<vi>, error out=w332:errorcluster)
          }
          frame Enabled {
          }
        }
        n94 = Add(x=w295, y=w294) -> (x+y=w296:dbl)
        n95 = Add(x=w294, y=w298) -> (x+y=w297:dbl)
        n96 = disable-structure shown="Enabled" {
          disable-tunnel: w306 -> [w327 w328]
          disable-tunnel: [w326 w328] -> w305
          disable-tunnel: w299 -> [w325 _]
          disable-tunnel: w303 -> [w324 w329]
          disable-tunnel: [w323 w329] -> w302
          disable-tunnel: w296 -> [w322 _]
          disable-tunnel: w297 -> [w321 _]
          frame Disabled {
            n97 = property class="XYGraph (strict)"(reference=w324, error in=w327, "ActYScl"=w325, "YScale.Maximum"=w322, "YScale.Minimum"=w321) -> (reference out=w323:refnum<vi>, error out=w326:errorcluster)
          }
          frame Enabled {
          }
        }
        n98 = local write "Plot Data"(w293) -> ()
      }
      frame "Update Channel" {
        n99 = for {
          tunnel: w381 -> [w490]
          tunnel: w357 -> [w491] mode=indexing
          tunnel: [w490] -> w355
          tunnel: [w489] -> w380 mode=indexing
          n100 = Unbundle By Name(w491) -> ("Channel name"=w489:string)
        }
        n101 = Search 1D Array(1D array=w380, element=w379) -> (index of element=w351:i32)  [unwired: 1 in]
        n102 = case shown="-1" w351 {
          selector: w351 -> [w382 w383]
          tunnel: [w382 w383] -> _
          frame 0, Default {
          }
          frame -1 {
          }
        }
        n103 = Index Array(array=w357, index=w351) -> (element=w358:T1)
        n104 = Unbundle By Name(w358) -> ("Value (original)"=w378:dbl[])
        n105 = Unbundle By Name(w358) -> ("Time (ms)"=w376:dbl[])
        n106 = Build Array (concatenate)(w378, w377) -> (w362:dbl[])
        n107 = Build Array (concatenate)(w376, w347) -> (w375:dbl[])
        n108 = Bundle By Name(cluster=w358, "Value (original)"=w362, "Time (ms)"=w375) -> (w359:T1)
        n109 = Replace Array Subset(array=w357, new element=w359, index=w351) -> (w356:T1[])
        n110 = flat-sequence {
          tunnel: w356 -> [w488]
          tunnel: [w488] -> w364
          tunnel: w355 -> [w487]
          tunnel: [w487] -> w374
          tunnel: [w486] -> _
          tunnel: w347 -> [w485]
          tunnel: [w485] -> w343
          frame #0 {
            n111 = Tick Count (ms)() -> (millisecond timer value=w486:u32)
          }
        }
        n112 = Subtract(x=w343, y=w345) -> (x-y=w344:dbl)
        n113 = Subtract(x=w343, y=w340) -> (x-y=w341:dbl)
        n114 = Greater Or Equal?(x=w344, y=w346) -> (x >= y?=w352:bool)
        n115 = Greater Or Equal?(x=w341, y=w342) -> (x >= y?=w363:bool)
        n116 = Not Equal?(x=-1, y=w351) -> ()  [unwired: 1 out]
        n117 = And(x=w352, y=TRUE) -> (x .and. y?=w349:bool)
        n118 = case shown="True" w349 {
          tunnel: w374 -> [w385 w412]
          tunnel: w373 -> [w391 w409]
          tunnel: w354 -> [w390 w410]
          tunnel: w342 -> [w389 w403]
          tunnel: w340 -> [w387 w396]
          tunnel: w357 -> [_ _]
          tunnel: [w384 w408] -> w372
          tunnel: [w391 w407] -> w371
          tunnel: [w390 w405] -> w370
          tunnel: [w389 w401] -> w369
          tunnel: w346 -> [w388 w402]
          tunnel: [w388 w400] -> w368
          tunnel: [w387 w398] -> w367
          tunnel: w345 -> [w386 _]
          tunnel: [w386 w399] -> w366
          tunnel: [w385 w404] -> w365
          tunnel: w364 -> [w384 w394]
          tunnel: w363 -> [_ w411]
          tunnel: w360 -> [_ w395]
          tunnel: w351 -> [_ w393]
          tunnel: w343 -> [_ w392]
          frame False {
            # "No need to update plot"
          }
          frame True {
            # "Update plot data when update timer > update time interval"
            n119 = for {
              tunnel: w412 -> [w481]
              tunnel: w394 -> [w484] mode=indexing
              tunnel: [w481] -> w406
              tunnel: [w480] -> w397 mode=indexing
              n120 = Unbundle By Name(w484) -> ("Value (original)"=w479:dbl[], "Time (ms)"=w482:dbl[])
              n121 = Bundle By Name(cluster=cluster{"Value":dbl[], "Time (ms)":dbl[]} {"Value"=[], "Time (ms)"=[]}, "Time (ms)"=w479, "Value"=w482) -> (w480:cluster{"Value":dbl[], "Time (ms)":dbl[]})
            }
            n122 = case shown="True" w411 {
              tunnel: w410 -> [w414 w445]
              tunnel: w409 -> [w423 w450]
              tunnel: w394 -> [_ w443]
              tunnel: [w424 w456] -> w408
              tunnel: [w423 w450] -> w407
              tunnel: w406 -> [w425 w455]
              tunnel: [w415 w452] -> w405
              tunnel: [w418 w451] -> w404
              tunnel: w403 -> [w422 w448]
              tunnel: w402 -> [w421 w449]
              tunnel: [w422 w448] -> w401
              tunnel: [w421 w449] -> w400
              tunnel: [w413 w431] -> w399
              tunnel: [w420 w431] -> w398
              tunnel: w394 -> [w424 _]
              tunnel: w397 -> [w417 _]
              tunnel: w396 -> [w420 _]
              tunnel: w395 -> [_ w446]
              tunnel: w393 -> [_ w444]
              tunnel: w392 -> [w413 w431]
              frame False {
                n123 = property class="XYGraph (strict)"(reference=w414, error in=w425, "Value"=w417) -> (reference out=w416:refnum<vi>, error out=w419:errorcluster)
                n124 = for {
                  tunnel: w419 -> [w430]
                  tunnel: [w428] -> w418
                  tunnel: w417 -> [_] mode=indexing
                  shift-right: [w426] -> w415
                  shift-left: w416 -> [w429]
                  i -> [w427]
                  n125 = property class="XYGraph (strict)"(reference=w429, error in=w430, "Active Plot"=w427, "Plot.YScaleIdx"=w427) -> (reference out=w426:refnum<vi>, error out=w428:errorcluster)
                }
              }
              frame True {
                n126 = To Double Precision Float(number=w446) -> ()  [unwired: 1 out]
                n127 = Add(x=w431, y=w448) -> (x+y=w447:dbl)
                n128 = for {
                  tunnel: w443 -> [w459] mode=indexing
                  tunnel: [w458] -> w442 mode=indexing
                  tunnel: [w457] -> w438 mode=indexing
                  n129 = Unbundle By Name(w459) -> ("Maximum"=w458:dbl, "Minimum"=w457:dbl)
                }
                n130 = Add Array Elements(numeric array=w442) -> (sum=w441:dbl)
                n131 = Add Array Elements(numeric array=w438) -> (sum=w440:dbl)
                n132 = Array Size(array=w438) -> (size(s)=w437:i32)
                n133 = Add(x=w441, y=w440) -> (x+y=w439:dbl)
                n134 = To Double Precision Float(number=w437) -> (double precision float=w436:dbl)
                n135 = Multiply(x=2.0, y=w436) -> (x*y=w434:dbl)
                n136 = Divide(x=w439, y=w434) -> (x/y=w433:dbl)
                n137 = for {
                  tunnel: w443 -> [w477] mode=indexing
                  tunnel: [w478] -> w456 mode=indexing
                  tunnel: w455 -> [w475]
                  tunnel: [w472] -> w454
                  tunnel: w447 -> [w465]
                  tunnel: w444 -> [w468]
                  tunnel: w433 -> [w467]
                  shift-right: [w466] -> w432
                  shift-left: w445 -> [w476]
                  tunnel: w431 -> [w464]
                  i -> [w460]
                  w469 = dbl[] [] ("Value (original)")
                  n138 = property class="XYGraph (strict)"(reference=w476, error in=w475, "XScale.Minimum"=w464, "XScale.Maximum"=w465, "Active Plot"=w468, "ActYScl"=w468) -> (reference out=w474:refnum<vi>, error out=w473:errorcluster)
                  n139 = Add(x=w465, y=w464) -> (x+y=w463:dbl)
                  n140 = Divide(x=w463, y=2.0) -> (x/y=w461:dbl)
                  n141 = Bundle By Name(cluster=T4 {"X"=0.0, "Y"=0.0} ("Cursor.Cursor Position"), "X"=w461, "Y"=w467) -> (w470:T4)
                  n142 = property class="XYGraph (strict)"(reference=w474, error in=w473, "Cursor.Cursor Position"=w470, "Cursor.Cursor Plot"=w460) -> (reference out=w466:refnum<vi>, error out=w472:errorcluster)
                  n143 = Bundle By Name(cluster=w477, "Value (original)"=w469, "Time (ms)"=w469) -> (w478:T1)
                }
                n144 = property class="XYGraph (strict)"(reference=w432, error in=w454, "Value"=cluster{"Value":dbl[], "Time (ms)":dbl[]}[] []) -> (reference out=w452:refnum<vi>, error out=w451:errorcluster)
              }
            }
          }
        }
      }
      frame "Get Cursor Data" {
        n145 = for {
          tunnel: w506 -> [w529]
          tunnel: [w529] -> w501
          tunnel: w502 -> [w528] mode=indexing
          tunnel: [w527] -> w505 mode=indexing
          n146 = Unbundle By Name(w528) -> ("Channel name"=w527:string)
        }
        n147 = Search 1D Array(1D array=w505, element=w504) -> (index of element=w503:i32)  [unwired: 1 in]
        n148 = Index Array(array=w502, index=w503) -> (element=w497:T1)
        n149 = Unbundle By Name(w497) -> ("Value (original)"=w496:dbl[])
        n150 = Unbundle By Name(w497) -> ("Time (ms)"=w500:dbl[])
        n151 = Array Size(array=w500) -> (size(s)=w499:i32)
        n152 = Decrement(x=w499) -> (x-1=w498:i32)
        n153 = for {
          N: w498 -> [_]
          tunnel: w501 -> [w526]
          tunnel: [w526] -> w495
          tunnel: w500 -> [w525]
          tunnel: w492 -> [w522]
          tunnel: w496 -> [w517]
          tunnel: [w515] -> w494
          i -> [w516]
          stop <- w518 stop-if-true
          n154 = Increment(x=w516) -> (x+1=w524:i32)
          n155 = Index Array(array=w525, index=w516) -> (element=w523:dbl)
          n156 = Index Array(array=w525, index=w524) -> (element=w521:dbl)
          n157 = Greater Or Equal?(x=w522, y=w523) -> (x >= y?=w520:bool)
          n158 = Less Or Equal?(x=w522, y=w521) -> (x <= y?=w519:bool)
          n159 = And(x=w520, y=w519) -> (x .and. y?=w518:bool)
          n160 = Index Array(array=w517, index=w516) -> (element=w515:dbl)
        }
        "Sample value" <- w494
        "Sample time (ms)" <- w492
      }
    }
  }
  "error out" <- w7
